vi "Get Power Sequence.vi"(11 "File Path":path) -> (1 "SMUs to Initialize (not in order)":T1[](array[typedef]), 2 "Power down Seq":T2[](array[typedef]) {"Power-down Seq" step=1; "Power-up Seq" step=1; "Wait Before Next (ms)" step=1; "Current Limit (A)" step=0.01 format="%.2g"; "Power-down Voltage (V)" step=0.01 format="%.2g"; "Power-up Voltage (V)" step=0.01 format="%.2g"}, 3 "Power up Seq":T2[](array[typedef]) {"Power-down Seq" step=1; "Power-up Seq" step=1; "Wait Before Next (ms)" step=1; "Current Limit (A)" step=0.01 format="%.2g"; "Power-down Voltage (V)" step=0.01 format="%.2g"; "Power-up Voltage (V)" step=0.01 format="%.2g"}, 5 "File Exists?":bool, 7 "Section Exists?":bool)   [LabVIEW 2023]
uses:
  DC Settings.ctl
  DC Ins Initialize.ctl
  <vilib>/Utility/file.llb/Read Delimited Spreadsheet (string).vi
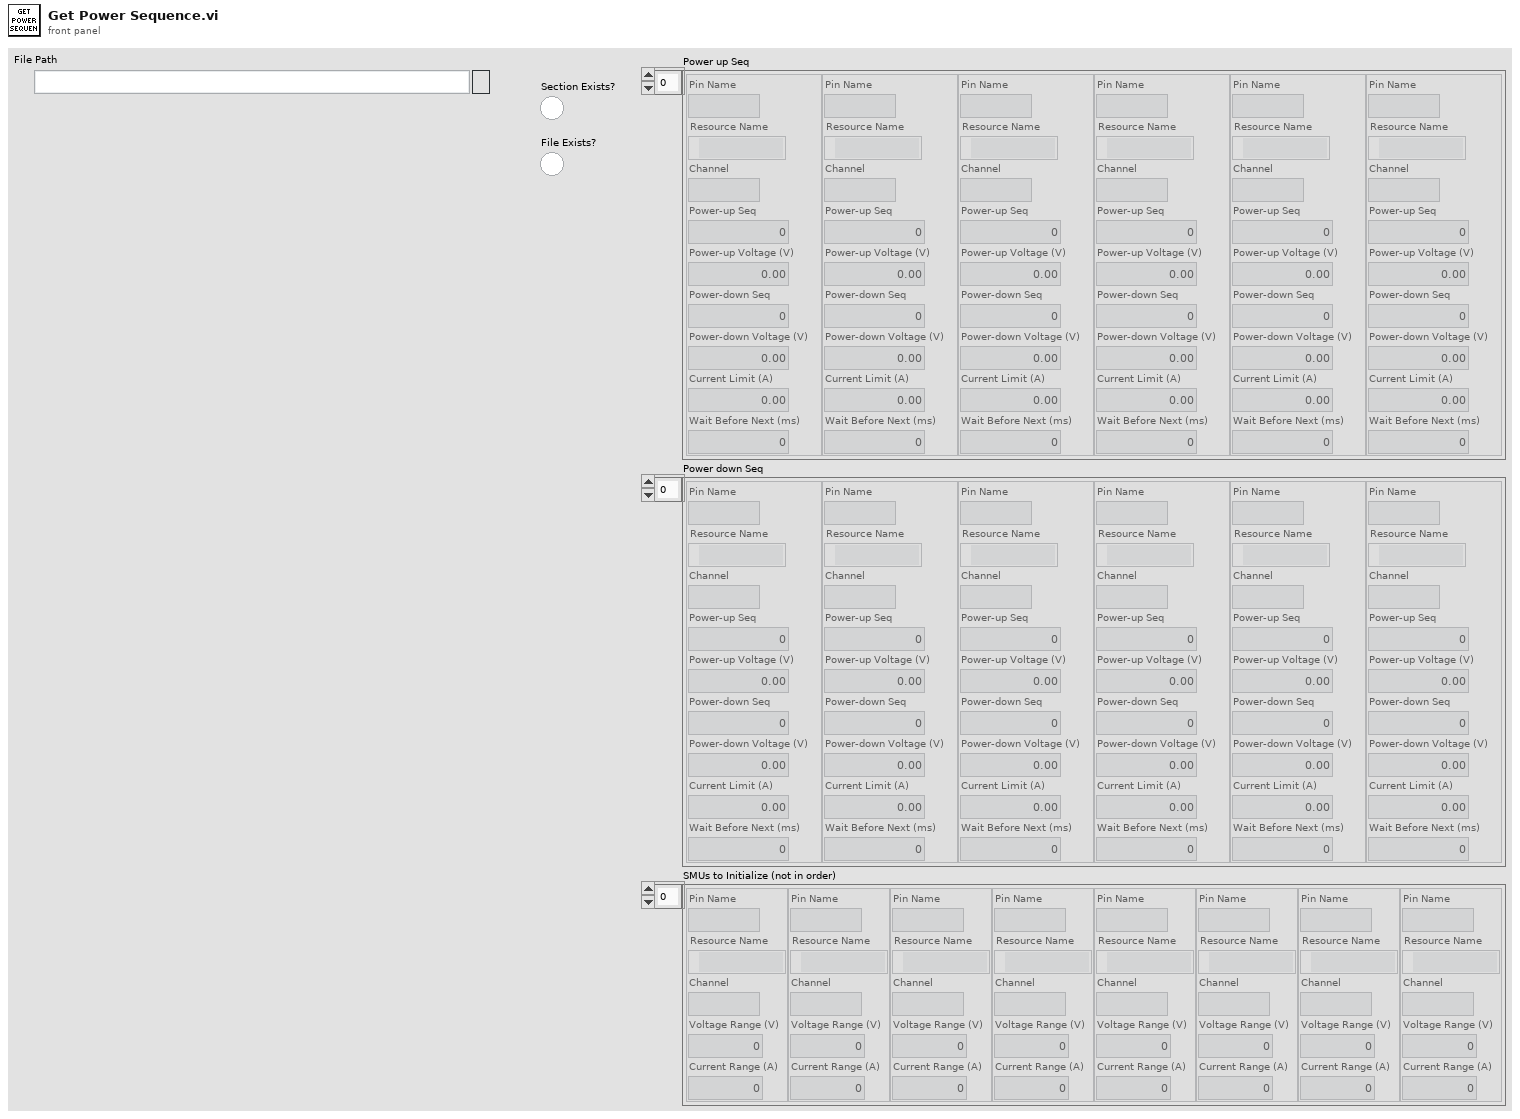
[diagram p1: front panel]
types:
  T1 = typedef "DC Ins Initialize.ctl" = cluster{"Pin Name":string, "Resource Name":refnum<k15>, "Channel":string, "Voltage Range (V)":dbl, "Current Range (A)":dbl}
  T2 = typedef "DC Settings.ctl" = cluster{"Pin Name":string, "Resource Name":refnum<k15>, "Channel":string, "Power-up Seq":u32, "Power-up Voltage (V)":dbl, "Power-down Seq":u32, "Power-down Voltage (V)":dbl, "Current Limit (A)":dbl, "Wait Before Next (ms)":u32}
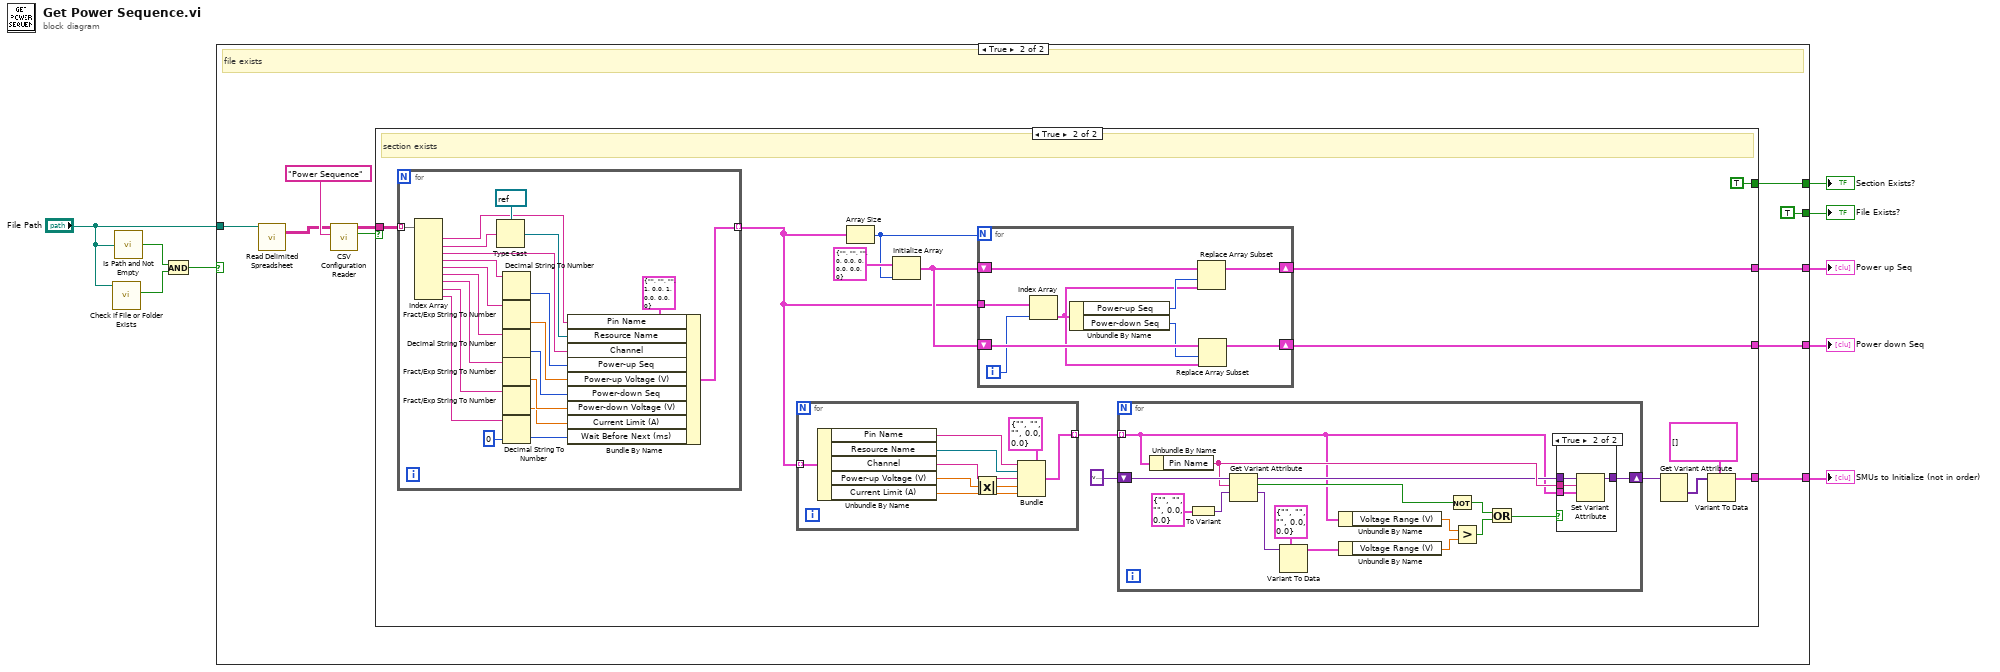
[diagram p0: block diagram]
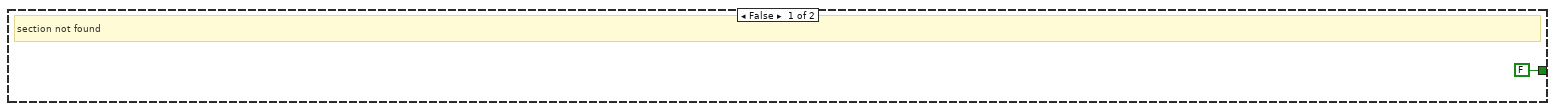
[diagram p3: hidden frame]
diagram:
  n1 = call <vilib>:"Check if File or Folder Exists.vi"("path"="File Path") -> ("file or folder exists?"=w3:bool)  [unwired: 8 in, 2 out]
  n2 = call <vilib>:"Is Path and Not Empty.vi"("path"="File Path") -> ("Is Path and Not Empty?"=w1:bool)  [unwired: 4 in]
  n3 = And(x=w1, y=w3) -> (x .and. y?=w4:bool)
  n4 = case shown="True" w4 {
    tunnel: "File Path" -> [_ w19]
    tunnel: [_ w18] -> w9
    tunnel: [_ w17] -> w8
    tunnel: [_ w16] -> w7
    tunnel: [_ TRUE] -> w6
    tunnel: [_ w10] -> w5
    frame False {
      # "file not found"
    }
    frame True {
      # "file exists"
      n5 = call-poly <vilib>:"Read Delimited Spreadsheet.vi"("file path (dialog if empty)"=w19) -> ("all rows"=w13:string[][])  [unwired: 9 in, 5 out]
      n6 = call "CSV Configuration Reader.vi"("Section"="Power Sequence" ("element"), "All CSV Configurations"=w13) -> ("Section Exists?"=w11:bool, "Extracted Configurations"=w12:string[][])  [unwired: 8 in]
      n7 = case shown="True" w11 {
        tunnel: [_ w30] -> w18
        tunnel: [_ w29] -> w17
        tunnel: [_ w23] -> w16
        tunnel: w12 -> [_ w22]
        tunnel: [FALSE TRUE] -> w10
        frame False {
          # "section not found"
        }
        frame True {
          # "section exists"
          n8 = for {
            tunnel: w22 -> [w55] mode=indexing
            tunnel: [w48] -> w31 mode=indexing
            n9 = Index Array(array=w55) -> (element #1=w38:string, element #2=w54:string, element #3=w36:string, element #4=w53:string, element #5=w43:string, element #6=w42:string, element #7=w44:string, element #8=w45:string, element #9=w46:string)  [unwired: 9 in]
            n10 = Type Cast(type=refnum<k15> refnum ("Resource Name"), x=w54) -> (*(type *) &x=w37:refnum<k15>)
            n11 = Decimal String To Number(string=w53) -> (number=w40:i32)  [unwired: 2 in, 1 out]
            n12 = Fract/Exp String To Number(string=w43) -> (number=w41:dbl)  [unwired: 3 in, 1 out]
            n13 = Decimal String To Number(string=w42) -> (number=w39:i32)  [unwired: 2 in, 1 out]
            n14 = Fract/Exp String To Number(string=w44) -> (number=w52:dbl)  [unwired: 3 in, 1 out]
            n15 = Fract/Exp String To Number(string=w45) -> (number=w51:dbl)  [unwired: 3 in, 1 out]
            n16 = Decimal String To Number(string=w46, default (0L)=u32 0 ("default (0 I32)")) -> (number=w50:u32)  [unwired: 1 in, 1 out]
            n17 = Bundle By Name(cluster=T2 {"Pin Name"="", "Resource Name"="", "Channel"="", "Power-up Seq"=1, "Power-up Voltage (V)"=0.0, "Power-down Seq"=1, "Power-down Voltage (V)"=0.0, "Current Limit (A)"=0.0, "Wait Before Next (ms)"=0} ("Pin Config"), "Pin Name"=w38, "Resource Name"=w37, "Channel"=w36, "Power-up Seq"=w40, "Power-up Voltage (V)"=w41, "Power-down Seq"=w39, "Power-down Voltage (V)"=w52, "Current Limit (A)"=w51, "Wait Before Next (ms)"=w50) -> (w48:T2)
          }
          n18 = for {
            tunnel: w31 -> [w85] mode=indexing
            tunnel: [w81] -> w24 mode=indexing
            n19 = Unbundle By Name(w85) -> ("Pin Name"=w84:string, "Resource Name"=w83:refnum<k15>, "Channel"=w82:string, "Power-up Voltage (V)"=w79:dbl, "Current Limit (A)"=w78:dbl)
            n20 = Absolute Value(x=w79) -> (abs(x)=w77:dbl)
            n21 = Bundle(cluster=T1 {"Pin Name"="", "Resource Name"="", "Channel"="", "Voltage Range (V)"=0.0, "Current Range (A)"=0.0}, "Pin Name"=w84, "Resource Name"=w83, "Channel"=w82, "Voltage Range (V)"=w77, "Current Range (A)"=w78) -> (w81:T1)
          }
          n22 = Array Size(array=w31) -> (size(s)=w33:i32)
          n23 = Initialize Array(T2 {"Pin Name"="", "Resource Name"="", "Channel"="", "Power-up Seq"=0, "Power-up Voltage (V)"=0.0, "Power-down Seq"=0, "Power-down Voltage (V)"=0.0, "Current Limit (A)"=0.0, "Wait Before Next (ms)"=0} ("Pin Config"), w33) -> (w32:T2[])
          n24 = for {
            N: w33 -> [_]
            shift-right: [w91] -> w30
            shift-left: w32 -> [w93]
            tunnel: w31 -> [w94]
            shift-right: [w89] -> w29
            shift-left: w32 -> [w90]
            i -> [w86]
            n25 = Index Array(array=w94, index=w86) -> (element=w87:T2)
            n26 = Unbundle By Name(w87) -> ("Power-up Seq"=w92:u32, "Power-down Seq"=w88:u32)
            n27 = Replace Array Subset(array=w93, new element=w87, index=w92) -> (w91:T2[])
            n28 = Replace Array Subset(array=w90, new element=w87, index=w88) -> (w89:T2[])
          }
          n29 = for {
            tunnel: w24 -> [w56] mode=indexing
            shift-right: [w71] -> w27
            shift-left: variant -> [w70]
            n30 = Unbundle By Name(w56) -> ("Pin Name"=w69:string)
            n31 = To Variant(anything=T1 {"Pin Name"="", "Resource Name"="", "Channel"="", "Voltage Range (V)"=0.0, "Current Range (A)"=0.0} ("Pin Config")) -> (Variant=w61:variant)
            n32 = Get Variant Attribute(Variant=w70, name=w69, default value (empty Variant)=w61) -> (duplicate Variant=w67:variant, found=w58:bool, value=w66:variant)  [unwired: 1 in, 1 out]
            n33 = Variant To Data(type=T1 {"Pin Name"="", "Resource Name"="", "Channel"="", "Voltage Range (V)"=0.0, "Current Range (A)"=0.0} ("Pin Config"), Variant=w66) -> (data=w65:T1)  [unwired: 1 in, 1 out]
            n34 = Unbundle By Name(w56) -> ("Voltage Range (V)"=w64:dbl)
            n35 = Unbundle By Name(w65) -> ("Voltage Range (V)"=w63:dbl)
            n36 = Not(x=w58) -> (.not. x?=w57:bool)
            n37 = Greater?(x=w64, y=w63) -> (0:w59:bool)
            n38 = Or(x=w57, y=w59) -> (x .or. y?=w60:bool)
            n39 = case shown="True" w60 {
              tunnel: [w72 w76] -> w71
              tunnel: w69 -> [_ w75]
              tunnel: w67 -> [w72 w74]
              tunnel: w56 -> [_ w73]
              frame False {
              }
              frame True {
                n40 = Set Variant Attribute(Variant=w74, name=w75, value=w73) -> (Variant out=w76:variant)  [unwired: 1 in, 2 out]
              }
            }
          }
          n41 = Get Variant Attribute(Variant=w27) -> (values=w26:variant[])  [unwired: 3 in, 3 out]
          n42 = Variant To Data(type=T1[] [] ("Array"), Variant=w26) -> (data=w23:T1[])  [unwired: 1 in, 1 out]
        }
      }
    }
  }
  "Power up Seq" <- w9
  "Power down Seq" <- w8
  "SMUs to Initialize (not in order)" <- w7
  "File Exists?" <- w6
  "Section Exists?" <- w5
